vi "Check for completed line.vi"(8 "error in (no error)":errorcluster caption="entrée d'erreur (pas d'erreur)", 11 "Game Board en entrée":refnum<class "Game Board.lvclass">) -> (0 "error out":errorcluster caption="sortie d'erreur", 3 "Game Board en sortie":refnum<class "Game Board.lvclass">)   [LabVIEW 2017, in "Game Board.lvclass"]
uses:
  Game Board.lvclass
  Game Board.lvclass/Game Board.ctl
  Wall_class/Wall.lvclass
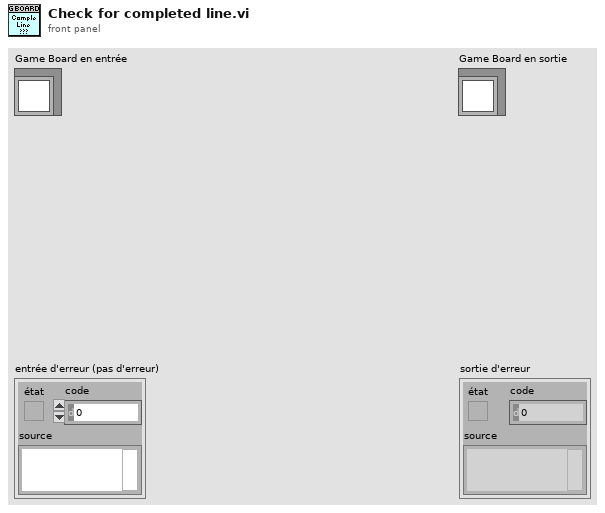
[diagram p1: front panel]
types:
  T1 = typedef "Coordinates.ctl" = cluster{"X":i32, "Y":i32}
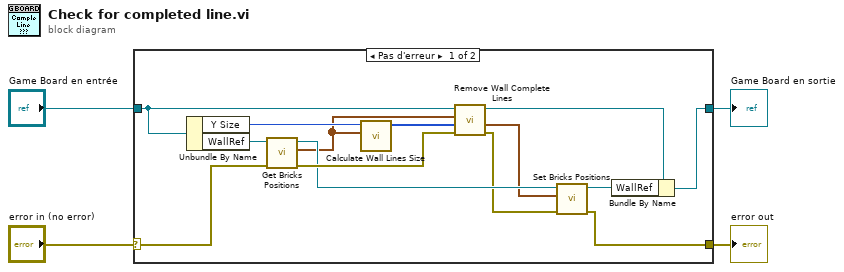
[diagram p0: block diagram]
diagram:
  n1 = case shown="Pas d'erreur" "error in (no error)" {
    selector: "error in (no error)" -> [w17 w20]
    tunnel: [w12 w20] -> w3
    tunnel: [w16 w19] -> w1
    tunnel: "Game Board en entrée" -> [w15 w19]
    frame No Error {
      n2 = Unbundle By Name(w15) -> ("Y Size"=w8:i32, "WallRef"=w18:refnum<class "Wall.lvclass">)
      n3 = call-dynamic "Get Bricks Positions.vi"("error in (no error)"=w17, "object in"=w18) -> ("error out"=w11:errorcluster, "Brick Wall"=w5:T1[], "object out"=w10:refnum<class "Wall.lvclass">)  [unwired: 7 in]
      n4 = call "Calculate Wall Lines Size.vi"("Brick Wall"=w5, "Y Size"=w8) -> ("Lines Size List"=w7:i32[])  [unwired: 9 in]
      n5 = call "Remove Wall Complete Lines.vi"("entrée d'erreur (pas d'erreur)"=w11, "Lines Size List"=w7, "Brick Wall In"=w5, "Game Board In"=w15) -> ("sortie d'erreur"=w6:errorcluster, "Brick Wall Out"=w9:T1[], "Game Board Out"=w14:refnum<class "Game Board.lvclass">)  [unwired: 5 in]
      n6 = call-dynamic "Set Bricks Positions.vi"("error in (no error)"=w6, "Brick Wall"=w9, "object in"=w10) -> ("error out"=w12:errorcluster, "object out"=w13:refnum<class "Wall.lvclass">)  [unwired: 7 in]
      n7 = Bundle By Name(cluster=w14, "WallRef"=w13) -> (w16:refnum<class "Game Board.lvclass">)
    }
    frame Error {
    }
  }
  "error out" <- w3
  "Game Board en sortie" <- w1
